vi "myRIO_BRig_RT_dataExp_Tcycle_Cue1_Audio_max.vi"() -> (2 "output_Tcycle_Cue1_Audio_max":i32)   [LabVIEW 2014]
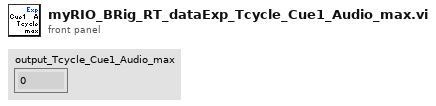
[diagram p1: front panel]
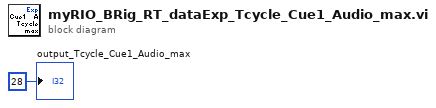
[diagram p0: block diagram]
diagram:
  "output_Tcycle_Cue1_Audio_max" <- 28 ("output_iBlock")
